vi "Easy Gabor Expansion.vi"(8 "error in (no error)":errorcluster, 11 "RefNum in":T1) -> (0 "error out":errorcluster, 2 "time waveform":dbl[](array[numeric]) format="%.2f", 3 "RefNum out":T1)   [LabVIEW 2017, in "SoundVib_Gabor.lvlib"]
doc: "Performs a simplified Gabor expansion on the Gabor coefficients referenced by <B>RefNum in</B> and returns the resulting 1D time waveform."
uses:
  <vilib>/addons/Sound and Vibration/Order Analysis/Gabor Order Tracking/SoundVib_Gabor.lvlib
  <vilib>/addons/Sound and Vibration/Order Analysis/Ref Gabor Order Tracking/GT RefNum.ctl
  <resource>/sndvib.dll
panel:
  # "Easy Gabor Expansion"
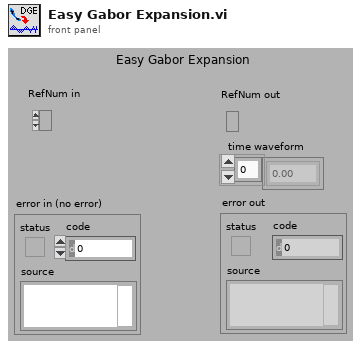
[diagram p1: front panel]
types:
  T1 = typedef "SoundVib_Gabor.lvlib/GT RefNum.ctl" = refnum<k1>
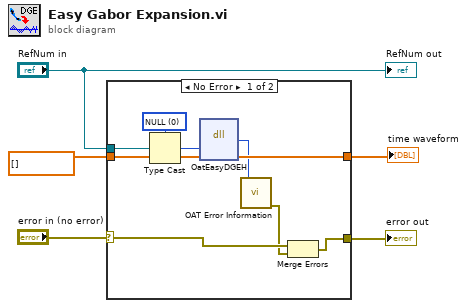
[diagram p0: block diagram]
diagram:
  n1 = case shown="No Error" "error in (no error)" {
    selector: "error in (no error)" -> [w8 w16]
    tunnel: [w6 w16] -> w5
    tunnel: "RefNum in" -> [w10 _]
    tunnel: [w12 w15] -> w2
    tunnel: dbl[] [] ("Time Series") -> [w9 w15]
    frame No Error {
      w14 = u32 0 items=["NULL"]
      n2 = Type Cast(type=w14, x=w10) -> (*(type *) &x=w13:u32)
      n3 = dll-call lib="C:/Program Files (x86)/National Instruments/LabVIEW 2017/resource/sndvib.*" fn="OatEasyDGEH"("refIn"=w13, "Time Series"=w9) -> ("return type"=w11:i32, "Time Series"=w12:dbl[])  [unwired: 4 in, 2 out]
      n4 = call <vilib>:"OAT Error Information.vi"("error code"=w11) -> ("error out"=w7:errorcluster)  [unwired: 6 in]
      n5 = Merge Errors(w8, w7) -> (w6:errorcluster)
    }
    frame Error {
    }
  }
  "error out" <- w5
  "time waveform" <- w2
  "RefNum out" <- "RefNum in"
